vi "Arma frase en Num (SubVI).vi"(9 "Posicion":i32, 10 "Direccion":i32, 11 "Codigo":u8[](array[numeric])) -> (3 "Codigo Completa":u8[](array[numeric]))   [LabVIEW 2014, in "CAP-USB.lvlib"]
uses:
  CAP-USB.lvlib
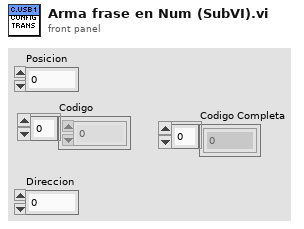
[diagram p1: front panel]
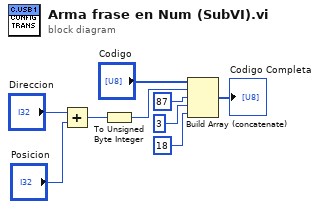
[diagram p0: block diagram]
diagram:
  n1 = Add(x="Direccion", y="Posicion") -> (x+y=w1:i32)
  n2 = To Unsigned Byte Integer(number=w1) -> (unsigned 8bit integer=w3:u8)
  n3 = Build Array (concatenate)("Codigo", w3, u8 87 ("f"), u8 3 ("f"), u8 18 ("f")) -> (→"Codigo Completa":u8[])
